vi "设置窗口.vi"() -> ()   [LabVIEW 2016]
uses:
  Holding Var.vi
panel:
  in  "布尔":bool
  in  "控制模式":enum16{"手动", "自动"}(ring)
  in  "关闭时间（H）":u16
  in  "开启时间（H）":u16
  in  "总开关":bool
  in  "选项卡控件":enum32{"氨氮", "总磷", "总氮", "CODMn", "CODcr"}(tab)
  in  "NH3N":T1={"水样测试"={"参数输入"={"采样模式"=enum."自动采样", "采样点数"=3, "变异系数设定值"=0.1, "重新取值百分比"=0.5, "偏差模式"=enum."相对偏差", "相对偏差百分比"=0.5, "绝对偏差值"=0.0}, "采样值"=[], "启用"=FALSE}, "零点核查"={"参数输入"={"采样模式"=enum."自动采样", "采样点数"=3, "变异系数设定值"=0.1, "重新取值百分比"=0.5, "偏差模式"=enum."相对偏差", "相对偏差百分比"=0.5, "绝对偏差值"=0.0}, "采样值"=[], "启用"=FALSE}, "跨度核查"={"参数输入"={"采样模式"=enum."自动采样", "采样点数"=3, "变异系数设定值"=0.1, "重新取值百分比"=0.5, "偏差模式"=enum."相对偏差", "相对偏差百分比"=0.5, "绝对偏差值"=0.0}, "采样值"=[], "启用"=FALSE}}
  in  "TP":T1={"水样测试"={"参数输入"={"采样模式"=enum."自动采样", "采样点数"=3, "变异系数设定值"=0.1, "重新取值百分比"=0.5, "偏差模式"=enum."相对偏差", "相对偏差百分比"=0.5, "绝对偏差值"=0.0}, "采样值"=[], "启用"=FALSE}, "零点核查"={"参数输入"={"采样模式"=enum."自动采样", "采样点数"=3, "变异系数设定值"=0.1, "重新取值百分比"=0.5, "偏差模式"=enum."相对偏差", "相对偏差百分比"=0.5, "绝对偏差值"=0.0}, "采样值"=[], "启用"=FALSE}, "跨度核查"={"参数输入"={"采样模式"=enum."自动采样", "采样点数"=3, "变异系数设定值"=0.1, "重新取值百分比"=0.5, "偏差模式"=enum."相对偏差", "相对偏差百分比"=0.5, "绝对偏差值"=0.0}, "采样值"=[], "启用"=FALSE}}
  in  "TN":T1={"水样测试"={"参数输入"={"采样模式"=enum."自动采样", "采样点数"=3, "变异系数设定值"=0.1, "重新取值百分比"=0.5, "偏差模式"=enum."相对偏差", "相对偏差百分比"=0.5, "绝对偏差值"=0.0}, "采样值"=[], "启用"=FALSE}, "零点核查"={"参数输入"={"采样模式"=enum."自动采样", "采样点数"=3, "变异系数设定值"=0.1, "重新取值百分比"=0.5, "偏差模式"=enum."相对偏差", "相对偏差百分比"=0.5, "绝对偏差值"=0.0}, "采样值"=[], "启用"=FALSE}, "跨度核查"={"参数输入"={"采样模式"=enum."自动采样", "采样点数"=3, "变异系数设定值"=0.1, "重新取值百分比"=0.5, "偏差模式"=enum."相对偏差", "相对偏差百分比"=0.5, "绝对偏差值"=0.0}, "采样值"=[], "启用"=FALSE}}
  in  "CODmn":T1={"水样测试"={"参数输入"={"采样模式"=enum."自动采样", "采样点数"=3, "变异系数设定值"=0.1, "重新取值百分比"=0.5, "偏差模式"=enum."相对偏差", "相对偏差百分比"=0.5, "绝对偏差值"=0.0}, "采样值"=[], "启用"=FALSE}, "零点核查"={"参数输入"={"采样模式"=enum."自动采样", "采样点数"=3, "变异系数设定值"=0.1, "重新取值百分比"=0.5, "偏差模式"=enum."相对偏差", "相对偏差百分比"=0.5, "绝对偏差值"=0.0}, "采样值"=[], "启用"=FALSE}, "跨度核查"={"参数输入"={"采样模式"=enum."自动采样", "采样点数"=3, "变异系数设定值"=0.1, "重新取值百分比"=0.5, "偏差模式"=enum."相对偏差", "相对偏差百分比"=0.5, "绝对偏差值"=0.0}, "采样值"=[], "启用"=FALSE}}
  in  "CODcr":T1={"水样测试"={"参数输入"={"采样模式"=enum."自动采样", "采样点数"=3, "变异系数设定值"=0.1, "重新取值百分比"=0.5, "偏差模式"=enum."相对偏差", "相对偏差百分比"=0.5, "绝对偏差值"=0.0}, "采样值"=[], "启用"=FALSE}, "零点核查"={"参数输入"={"采样模式"=enum."自动采样", "采样点数"=3, "变异系数设定值"=0.1, "重新取值百分比"=0.5, "偏差模式"=enum."相对偏差", "相对偏差百分比"=0.5, "绝对偏差值"=0.0}, "采样值"=[], "启用"=FALSE}, "跨度核查"={"参数输入"={"采样模式"=enum."自动采样", "采样点数"=3, "变异系数设定值"=0.1, "重新取值百分比"=0.5, "偏差模式"=enum."相对偏差", "相对偏差百分比"=0.5, "绝对偏差值"=0.0}, "采样值"=[], "启用"=FALSE}}
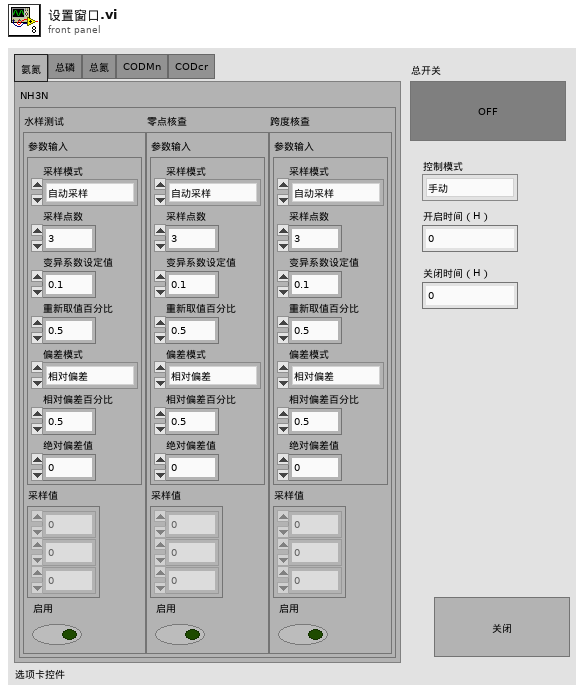
[diagram p1: front panel]
types:
  T1 = cluster{"水样测试":cluster{"参数输入":cluster{"采样模式":enum16{"自动采样", "手动采样"}, "采样点数":i32, "变异系数设定值":dbl, "重新取值百分比":dbl, "偏差模式":enum16{"相对偏差", "绝对偏差"}, "相对偏差百分比":dbl, "绝对偏差值":dbl}, "采样值":dbl[], "启用":bool}, "零点核查":cluster{"参数输入":cluster{"采样模式":enum16{"自动采样", "手动采样"}, "采样点数":i32, "变异系数设定值":dbl, "重新取值百分比":dbl, "偏差模式":enum16{"相对偏差", "绝对偏差"}, "相对偏差百分比":dbl, "绝对偏差值":dbl}, "采样值":dbl[], "启用":bool}, "跨度核查":cluster{"参数输入":cluster{"采样模式":enum16{"自动采样", "手动采样"}, "采样点数":i32, "变异系数设定值":dbl, "重新取值百分比":dbl, "偏差模式":enum16{"相对偏差", "绝对偏差"}, "相对偏差百分比":dbl, "绝对偏差值":dbl}, "采样值":dbl[], "启用":bool}}
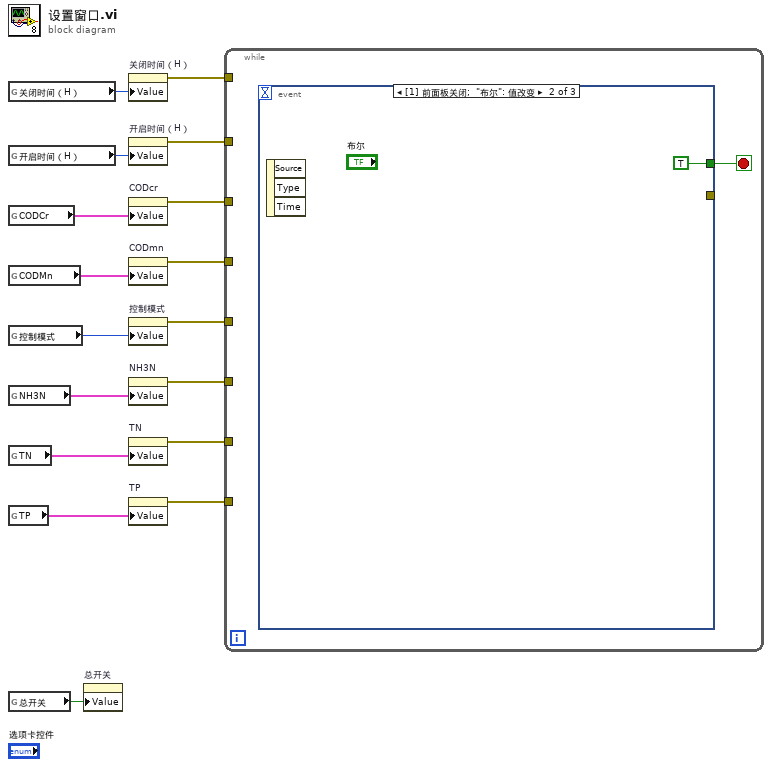
[diagram p0: block diagram]
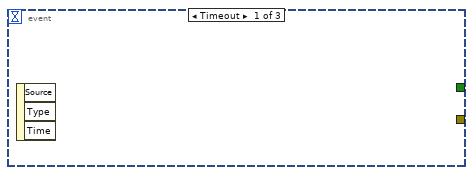
[diagram p2: hidden frame]
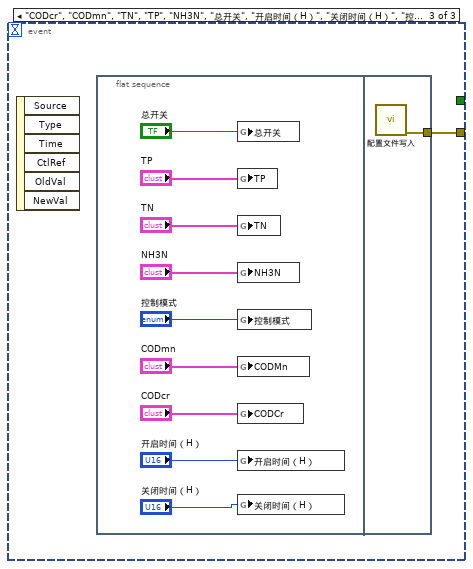
[diagram p3: hidden frame]
diagram:
  n1 = global read "Holding Var.vi" "关闭时间（H）"() -> (w9:u16)
  n2 = global read "Holding Var.vi" "开启时间（H）"() -> (w10:u16)
  n3 = global read "Holding Var.vi" "CODCr"() -> (w11:T1)
  n4 = global read "Holding Var.vi" "CODMn"() -> (w12:T1)
  n5 = global read "Holding Var.vi" "控制模式"() -> (w13:enum16{"手动", "自动"})
  n6 = global read "Holding Var.vi" "NH3N"() -> (w14:T1)
  n7 = global read "Holding Var.vi" "TN"() -> (w15:T1)
  n8 = global read "Holding Var.vi" "TP"() -> (w16:T1)
  n9 = global read "Holding Var.vi" "总开关"() -> (w17:bool)
  n10 = property on="总开关" class="Bool (严格)"("Value"=w17) -> ()  [unwired: 2 in, 2 out]
  n11 = property on="关闭时间（H）" class="DigNum (严格)"("Value"=w9) -> (error out=w1:errorcluster)  [unwired: 2 in, 1 out]
  n12 = property on="开启时间（H）" class="DigNum (严格)"("Value"=w10) -> (error out=w2:errorcluster)  [unwired: 2 in, 1 out]
  n13 = property on="CODcr" class="Clust (严格)"("Value"=w11) -> (error out=w3:errorcluster)  [unwired: 2 in, 1 out]
  n14 = property on="CODmn" class="Clust (严格)"("Value"=w12) -> (error out=w4:errorcluster)  [unwired: 2 in, 1 out]
  n15 = property on="控制模式" class="Enum (严格)"("Value"=w13) -> (error out=w5:errorcluster)  [unwired: 2 in, 1 out]
  n16 = property on="NH3N" class="Clust (严格)"("Value"=w14) -> (error out=w6:errorcluster)  [unwired: 2 in, 1 out]
  n17 = property on="TN" class="Clust (严格)"("Value"=w15) -> (error out=w7:errorcluster)  [unwired: 2 in, 1 out]
  n18 = property on="TP" class="Clust (严格)"("Value"=w16) -> (error out=w8:errorcluster)  [unwired: 2 in, 1 out]
  n19 = while {
    tunnel: w8 -> [_]
    tunnel: w7 -> [_]
    tunnel: w6 -> [_]
    tunnel: w5 -> [_]
    tunnel: w4 -> [_]
    tunnel: w3 -> [_]
    tunnel: w2 -> [_]
    tunnel: w1 -> [_]
    stop <- w18 stop-if-true
    n20 = event shown="[1] 前面板关闭;  \"布尔\": 值改变" {
      selector: _ -> [_ _ _]
      dyn-events: _ -> [_ _ _]
      timeout: _ -> [_ _ _]
      tunnel: [_ TRUE _] -> w18
      tunnel: [_ _ w20] -> _
      event Timeout {
        n21 = event-data() -> ()  [unwired: 1 in, 3 out]
      }
      event Panel Close; "布尔": Value Change {
        n22 = event-data() -> ()  [unwired: 1 in, 3 out]
      }
      event "CODcr", "CODmn", "TN", "TP", "NH3N", "总开关", "开启时间（H）", "关闭时间（H）", "控制模式": Value Change {
        n23 = event-data() -> ()  [unwired: 1 in, 6 out]
        n24 = flat-sequence {
          tunnel: [w30] -> w20
          frame #0 {
            n25 = global write "Holding Var.vi" "总开关"("总开关") -> ()
            n26 = global write "Holding Var.vi" "TP"("TP") -> ()
            n27 = global write "Holding Var.vi" "TN"("TN") -> ()
            n28 = global write "Holding Var.vi" "NH3N"("NH3N") -> ()
            n29 = global write "Holding Var.vi" "控制模式"("控制模式") -> ()
            n30 = global write "Holding Var.vi" "CODMn"("CODmn") -> ()
            n31 = global write "Holding Var.vi" "CODCr"("CODcr") -> ()
            n32 = global write "Holding Var.vi" "开启时间（H）"("开启时间（H）") -> ()
            n33 = global write "Holding Var.vi" "关闭时间（H）"("关闭时间（H）") -> ()
          }
          frame #1 {
            n34 = call "配置文件写入.vi"() -> ("错误输出"=w30:errorcluster)  [unwired: 11 in]
          }
        }
      }
    }
  }
